vi "Read T.vi"(8 "error in (no error)":errorcluster, 11 "M data in":refnum<class "M data.lvclass">) -> (0 "error out":errorcluster, 2 "T":sgl, 3 "M data out":refnum<class "M data.lvclass">)   [LabVIEW 2015, in "Alicat Lib.lvlib" / "M data.lvclass"]
uses:
  M data.lvclass
  M data.lvclass/M data.ctl
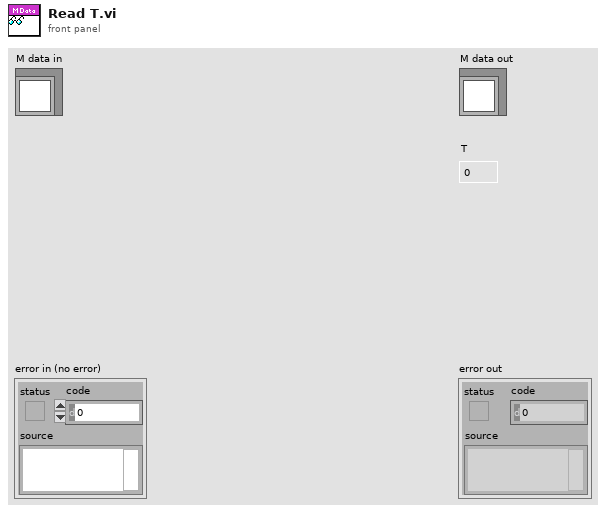
[diagram p1: front panel]
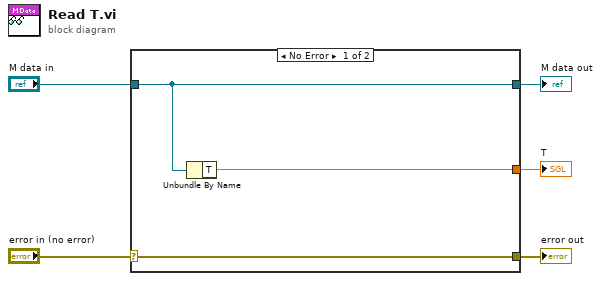
[diagram p0: block diagram]
diagram:
  n1 = case shown="No Error" "error in (no error)" {
    selector: "error in (no error)" -> [w8 w9]
    tunnel: [w8 w9] -> w4
    tunnel: [w7 w10] -> w2
    tunnel: "M data in" -> [w7 w10]
    tunnel: [w6 _] -> w1
    frame No Error {
      n2 = Unbundle By Name(w7) -> ("T"=w6:sgl)
    }
    frame Error {
    }
  }
  "error out" <- w4
  "M data out" <- w2
  "T" <- w1
